vi "EminemStateMachine.vi"(5 "EminemCommand":bool[](array[boolean]), 7 "EminemCancel":bool, 8 "LowerShoot_At_Speed":bool, 9 "UpperShoot_At_Speed":bool, 10 "LowerShoot_Speed_RPM":dbl=1.0 format="%#_13g", 11 "UpperShoot_Speed_RPM":dbl=4000.0 format="%#_13g") -> (0 "Box states":T1=enum."13-AmpDone", 1 "AmpAndFeed-MotorDmd":dbl, 2 "LowerShooter-RPM_Dmd":dbl, 3 "UpperShooterAndAmp-RPM_Dmd":dbl)   [LabVIEW 2023]
doc: "Process Intake State Machine"
uses:
  Intake/IntakeState.ctl
  EminemStatesEnum.ctl
  _UNUSED/EminemNoteState.ctl
  <vilib>/Rock Robotics/WPI/ThirdParty/JAS_Junk/TrajLib/Trajectory_Library.lvlib
  EminemGlobals.vi
panel:
  in  "ActualShooterSpd":dbl
  # "WHAT IS THIS ???"
  # "Click here to set min"
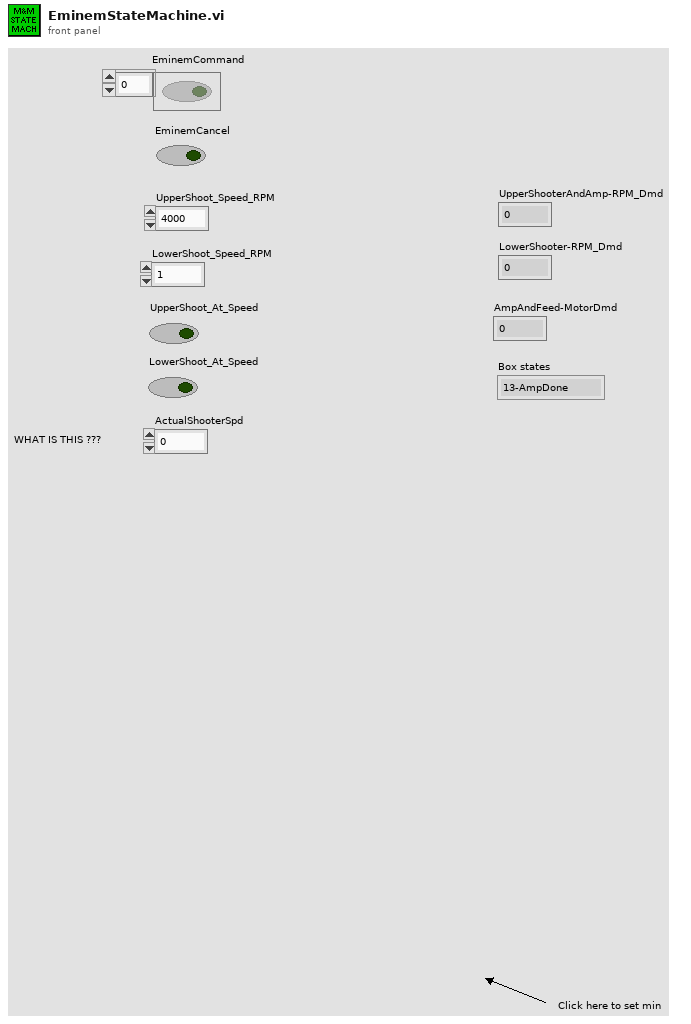
[diagram p1: front panel]
types:
  T1 = typedef "EminemStatesEnum.ctl" = enum16{"0-Init", "1-WaitForCmd", "2-Cancel", "3-ShootStart", "4-ShootRev", "5-ShootUpToSpd?", "6-ShootStartFeed&Timer", "7-ShootTimerOrSensorDone", "8-ShootDone", "9-AmpStart", "10-AmpUpToSpd?", "11-AmpStartFeed&Timer", "12-AmpTimerOrSensorDone", "13-AmpDone"}
  T2 = typedef "EminemNoteState.ctl" = enum16{"0-NoteInShooterWheels", "1-MisalignedNote", "2-NoNote", "3-HaveNote"}
  T3 = typedef "EminemStatesEnum.ctl" = enum16{"get input", "start shoot wheels", "up to speed?", "run intake", "have ring?", "stop intake and shooter", "start intake", "pick up ring or  _ sec?", "stop intake", "start source  intake", "pick up note?", "stop intake shooter", "shoot amp", "used note?", "stop amp intake", "initilization", "pre rev"}
  T4 = typedef "Trajectory_Library.lvlib/TIMER.ctl" = cluster{"StartTime":dbl, "Accumulated TIme":dbl, "Running":bool, "semaphore":T5}
  T5 = typedef "Semaphore RefNum" = refnum<k1>
  T6 = typedef "IntakeState.ctl" = enum16{"0-init", "1-cancel", "2-wait-for-cmd", "3-intake-check-for-note", "4-intake-start-intake", "5-intake-have-note-yet", "6-intake-stop-motor", "7-spit-out", "8-feed-note-to-shooter"}
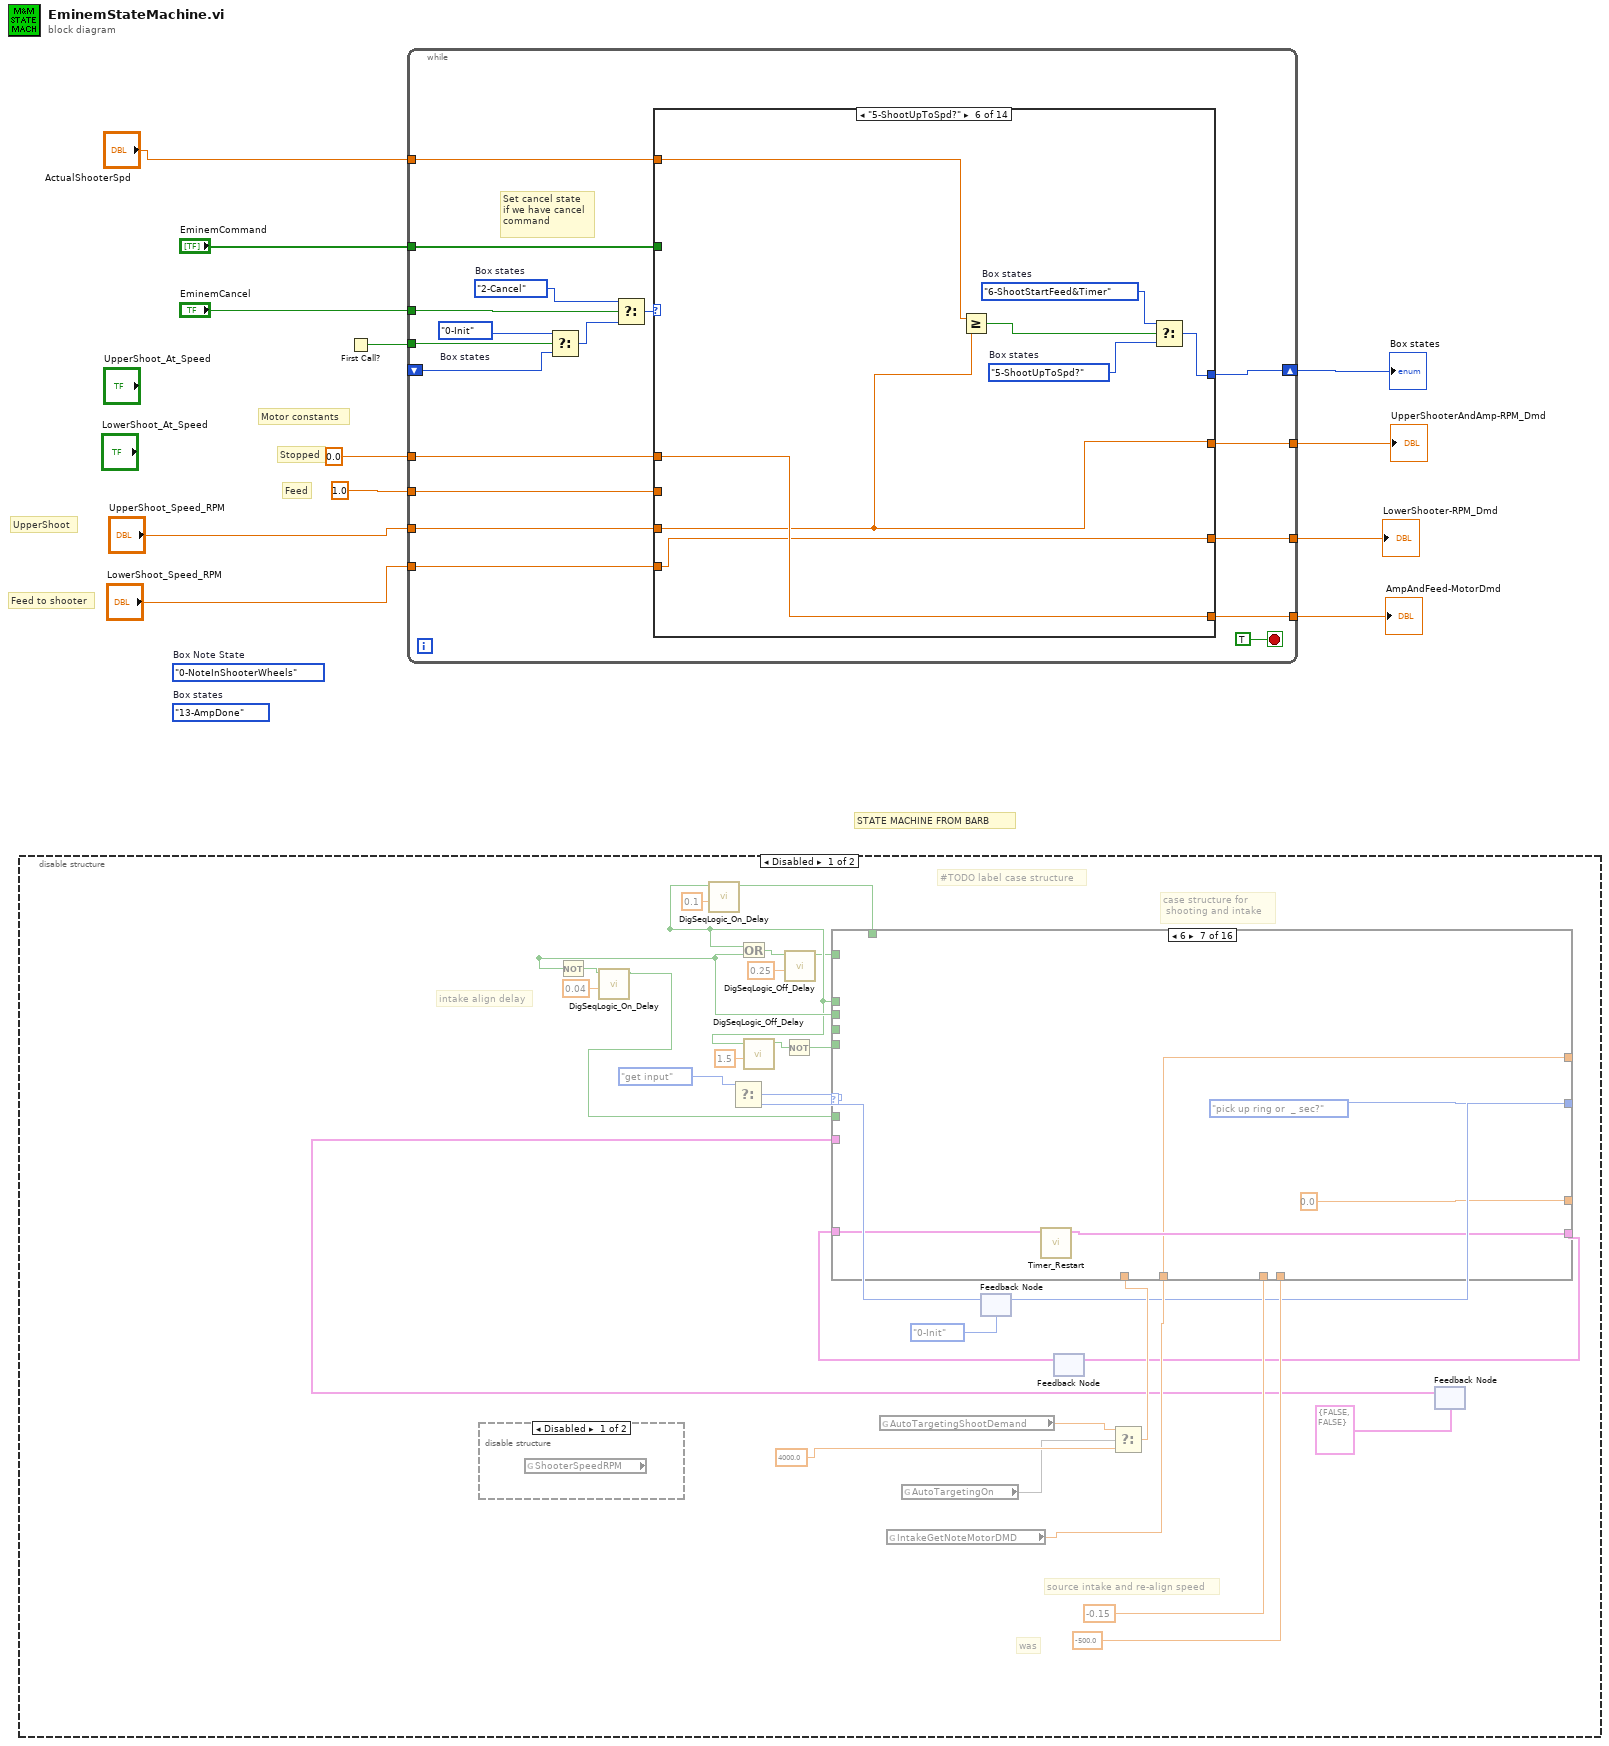
[diagram p0: block diagram]
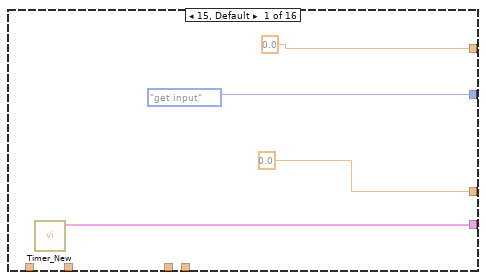
[diagram p3: hidden frame]
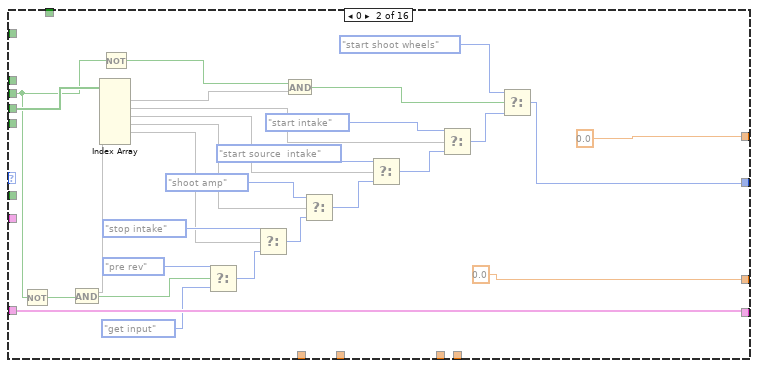
[diagram p4: hidden frame]
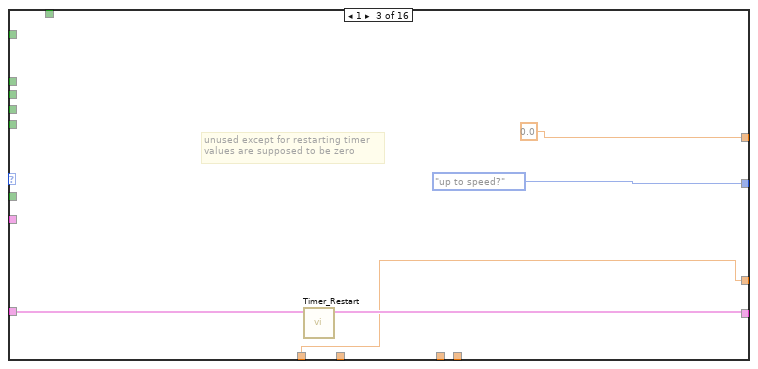
[diagram p5: hidden frame]
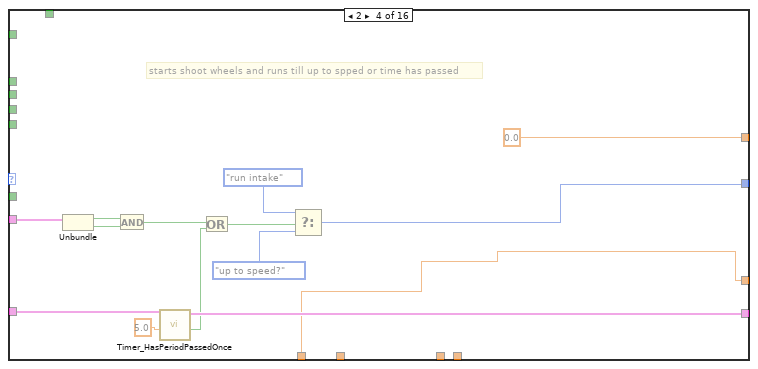
[diagram p6: hidden frame]
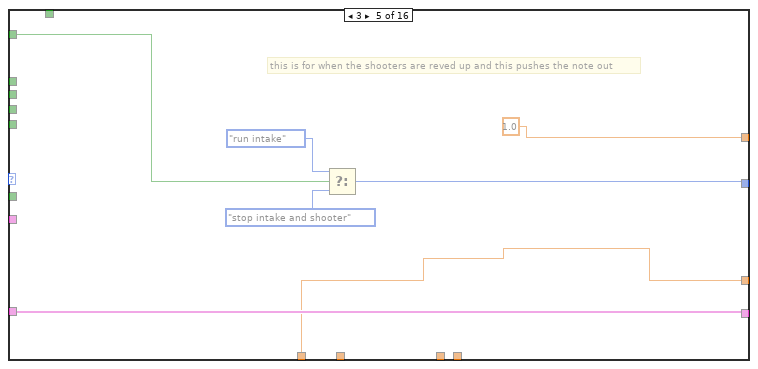
[diagram p7: hidden frame]
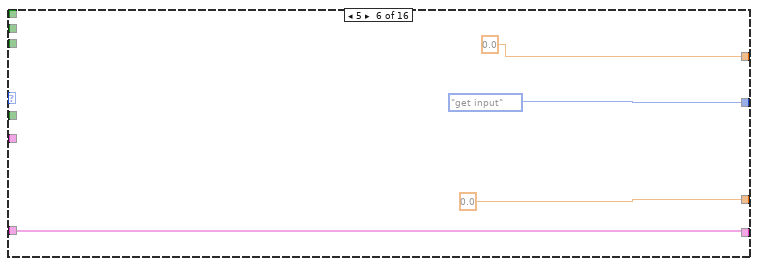
[diagram p8: hidden frame]
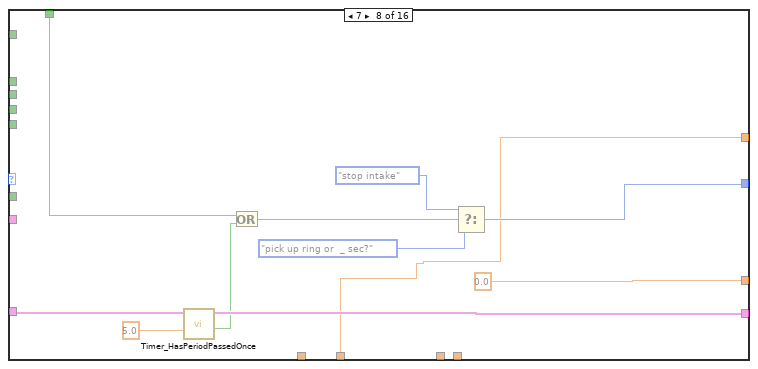
[diagram p9: hidden frame]
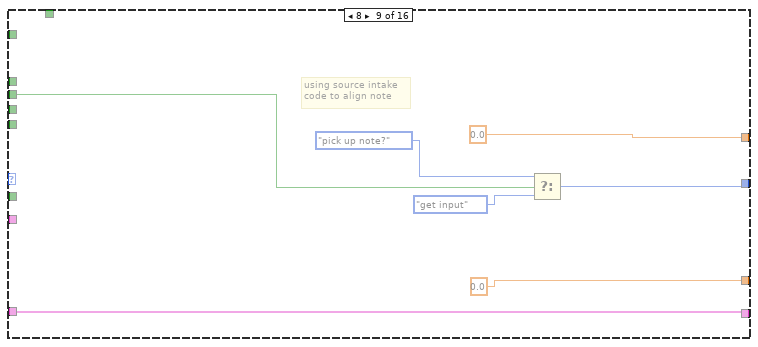
[diagram p10: hidden frame]
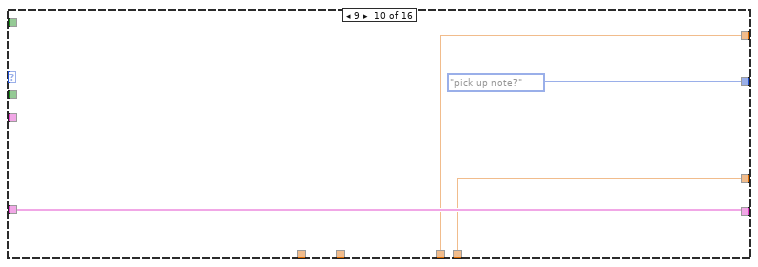
[diagram p11: hidden frame]
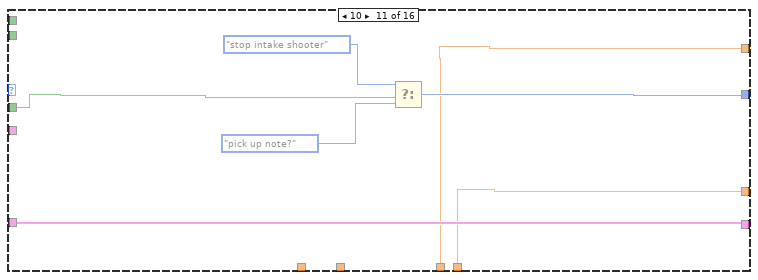
[diagram p12: hidden frame]
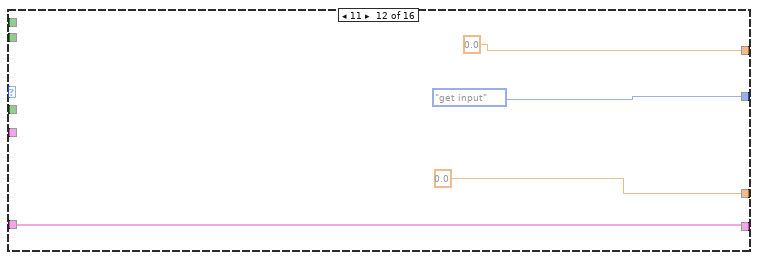
[diagram p13: hidden frame]
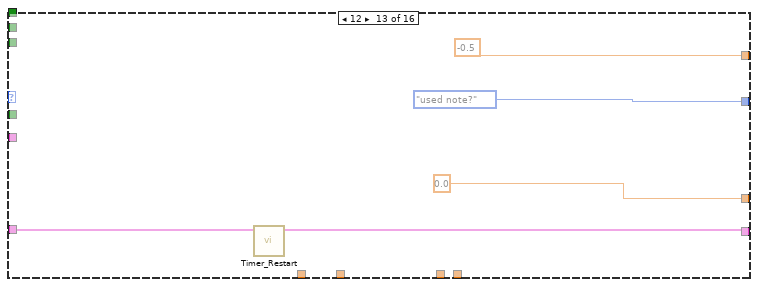
[diagram p14: hidden frame]
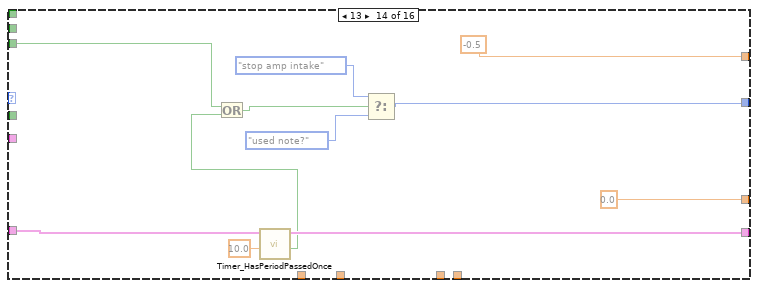
[diagram p15: hidden frame]
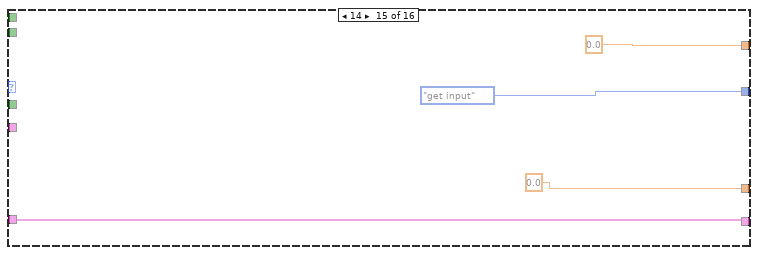
[diagram p16: hidden frame]
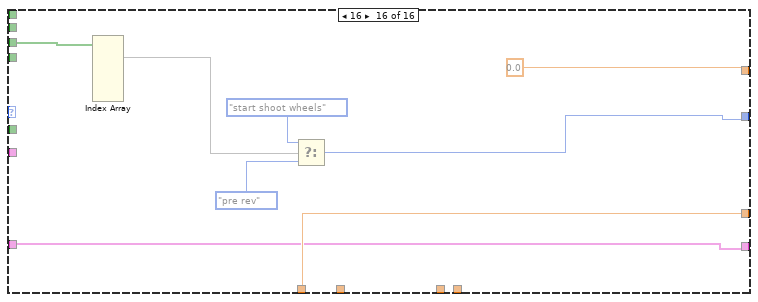
[diagram p17: hidden frame]
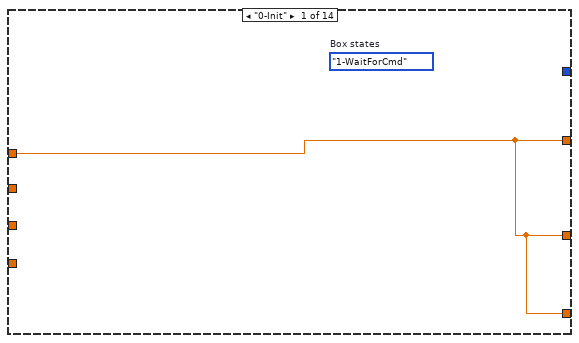
[diagram p19: hidden frame]
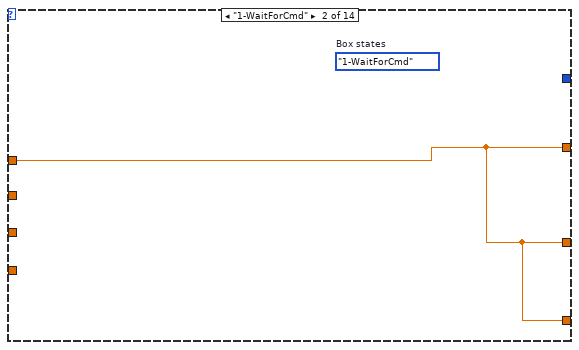
[diagram p20: hidden frame]
diagram:
  (unwired) EminemNoteState."0-NoteInShooterWheels"  # Box Note State
  (unwired) EminemStatesEnum."13-AmpDone"  # Box states
  # "STATE MACHINE FROM BARB"
  # "Feed to shooter"
  # "UpperShoot"
  # "Feed"
  # "Stopped"
  # "Motor constants"
  n1 = disable-structure shown="Disabled" {
    frame Disabled {
      # "intake align delay"
      # "was"
      # "source intake and re-align speed"
      # "#TODO label case structure"
      # "case structure for\n shooting and intake"
      n2 = disable-structure shown="Disabled" {
        frame Disabled {
          n3 = global read "EminemGlobals.vi" "ShooterSpeedRPM"() -> ()  [unwired: 1 out]
        }
        frame Enabled {
        }
      }
      n4 = global read "EminemGlobals.vi" "AutoTargetingShootDemand"() -> (w32:dbl)
      n5 = global read "EminemGlobals.vi" "IntakeGetNoteMotorDMD"() -> (w29:dbl)
      n6 = global read "EminemGlobals.vi" "AutoTargetingOn"() -> (w33)
      n7 = feedback #1(EminemStatesEnum."0-Init") -> (w38:u16)
      n8 = Select(t=EminemStatesEnum."get input" ("Box states"), f=w38) -> (s=w18:bool, s? t:f=w17:u16)
      n9 = feedback #2() -> (w22:T4)  [unwired: 1 in]
      n10 = Select(t=w32, s=w33, f=4000.0) -> (s? t:f=w34:dbl)
      n11 = feedback #3(cluster{bool, bool} {FALSE, FALSE}) -> (w15:cluster{bool, bool})
      n12 = feedback-in #3() -> ()  [unwired: 1 out]
      n13 = Not(x=w41) -> (.not. x?=w39:bool)
      n14 = call <vilib>:"DigSeqLogic_On_Delay.vi"("Delay"=0.04, "Input"=w39) -> ("Output"=w42:bool)  [unwired: 8 in, 1 out]
      n15 = call <vilib>:"DigSeqLogic_On_Delay.vi"("Delay"=0.1 ("On Delay Time\nSeconds"), "Input"=w35) -> ("Output"=w31:bool)  [unwired: 8 in, 1 out]
      n16 = Or(x=w35, y=w41) -> (x .or. y?=w24:bool)
      n17 = call <vilib>:"DigSeqLogic_Off_Delay.vi"("Delay"=0.25 ("Off Delay Tme\nSeconds"), "Input"=w24) -> ("Output"=w25:bool)  [unwired: 8 in, 1 out]
      n18 = call <vilib>:"DigSeqLogic_Off_Delay.vi"("Delay"=1.5 ("Off Delay Tme\nSeconds"), "Input"=w35) -> ("Output"=w27:bool)  [unwired: 8 in, 1 out]
      n19 = Not(x=w27) -> (.not. x?=w28:bool)
      n20 = case shown="6" w17 {
        tunnel: [EminemStatesEnum."get input" ("Box states") w69 EminemStatesEnum."up to speed?" ("Box states") w89 w98 EminemStatesEnum."get input" ("Box states") EminemStatesEnum."pick up ring or  _ sec?" ("Box states") w118 w125 EminemStatesEnum."pick up note?" ("Box states") w136 EminemStatesEnum."get input" ("Box states") EminemStatesEnum."used note?" ("Box states") w155 EminemStatesEnum."get input" ("Box states") w168] -> w14
        tunnel: w15 -> [_ _ _ w92 _ _ _ _ _ _ _ _ _ _ _ _]
        tunnel: [0.0 0.0 w76 w81 w95 0.0 0.0 0.0 0.0 w129 w134 0.0 0.0 0.0 0.0 w169] -> _
        tunnel: [0.0 0.0 0.0 0.0 1.0 0.0 w106 w112 0.0 w130 w135 0.0 -0.5 -0.5 0.0 0.0] -> _
        tunnel: [_ w74 _ _ _ _ _ _ _ _ _ _ _ _ _ w166] -> w16
        tunnel: [_ _ _ _ _ _ _ _ _ _ _ _ _ _ _ _] -> w35
        tunnel: [_ w51 _ _ _ _ _ _ w122 _ _ _ _ _ _ _] -> w41
        tunnel: [w44 w61 w77 w86 w97 w102 w108 w114 w126 w131 w139 w140 w144 w153 w160 w167] -> w21
        tunnel: w22 -> [_ w61 w78 w87 w97 w102 w107 w116 w126 w131 w139 w140 w145 w154 w160 w167]
        tunnel: w25 -> [_ _ _ _ w96 _ _ _ _ _ _ _ _ _ _ _]
        tunnel: w28 -> [_ _ _ _ _ _ _ _ _ _ _ _ _ w149 _ _]
        tunnel: w34 -> [_ _ w76 w81 w95 _ _ _ _ _ _ _ _ _ _ w169]
        tunnel: w29 -> [_ _ _ _ _ _ w106 w112 _ _ _ _ _ _ _ _]
        tunnel: w31 -> [_ _ _ _ _ _ _ w111 _ _ _ _ _ _ _ _]
        tunnel: -0.15 -> [_ _ _ _ _ _ _ _ _ w130 w135 _ _ _ _ _]
        tunnel: -500.0 -> [_ _ _ _ _ _ _ _ _ w129 w134 _ _ _ _ _]
        tunnel: w42 -> [_ _ _ _ _ _ _ _ _ _ w133 _ _ _ _ _]
        frame 15, Default {
          n21 = call <vilib>:"Timer_New.vi"() -> ("TIMER"=w44:T4)  [unwired: 11 in]
        }
        frame 0 {
          n22 = Not(x=w51) -> (.not. x?=w49:bool)
          n23 = Index Array(array=w74) -> (element #1=w59, element #2=w66, element #3=w65, element #4=w64, element #5=w55, element #6=w50)  [unwired: 6 in]
          n24 = And(x=w50, y=w49) -> (x .and. y?=w48:bool)
          n25 = Not(x=w51) -> (.not. x?=w58:bool)
          n26 = Select(t=EminemStatesEnum."pre rev" ("Box states"), s=w48, f=EminemStatesEnum."get input" ("Box states")) -> (s? t:f=w54:T3)
          n27 = Select(t=EminemStatesEnum."stop intake" ("Box states"), s=w55, f=w54) -> (s? t:f=w57:T3)
          n28 = And(x=w58, y=w59) -> (x .and. y?=w60:bool)
          n29 = Select(t=EminemStatesEnum."shoot amp" ("Box states"), s=w64, f=w57) -> (s? t:f=w70:T3)
          n30 = Select(t=EminemStatesEnum."start source  intake", s=w65, f=w70) -> (s? t:f=w71:T3)
          n31 = Select(t=EminemStatesEnum."start intake" ("Box states"), s=w66, f=w71) -> (s? t:f=w72:T3)
          n32 = Select(t=EminemStatesEnum."start shoot wheels" ("Box states"), s=w60, f=w72) -> (s? t:f=w69:T3)
        }
        frame 1 {
          # "unused except for restarting timer\nvalues are supposed to be zero"
          n33 = call <vilib>:"Timer_Restart.vi"("in Timer"=w78) -> ("out Timer"=w77:T4)  [unwired: 10 in]
        }
        frame 2 {
          # "starts shoot wheels and runs till up to spped or time has passed"
          n34 = Unbundle(w92) -> (w91:bool, w90:bool)
          n35 = And(x=w91, y=w90) -> (x .and. y?=w84:bool)
          n36 = call <vilib>:"Timer_HasPeriodPassedOnce.vi"("Period"=5.0, "in Timer"=w87) -> ("Expired"=w82:bool, "out Timer"=w86:T4)  [unwired: 7 in, 1 out]
          n37 = Or(x=w84, y=w82) -> (x .or. y?=w83:bool)
          n38 = Select(t=EminemStatesEnum."run intake" ("Box states"), s=w83, f=EminemStatesEnum."up to speed?" ("Box states")) -> (s? t:f=w89:T3)
        }
        frame 3 {
          # "this is for when the shooters are reved up and this pushes the note out"
          n39 = Select(t=EminemStatesEnum."run intake" ("Box states"), s=w96, f=EminemStatesEnum."stop intake and shooter" ("Box states")) -> (s? t:f=w98:T3)
        }
        frame 5 {
        }
        frame 6 {
          n40 = call <vilib>:"Timer_Restart.vi"("in Timer"=w107) -> ("out Timer"=w108:T4)  [unwired: 10 in]
        }
        frame 7 {
          n41 = call <vilib>:"Timer_HasPeriodPassedOnce.vi"("Period"=5.0, "in Timer"=w116) -> ("Expired"=w113:bool, "out Timer"=w114:T4)  [unwired: 7 in, 1 out]
          n42 = Or(x=w111, y=w113) -> (x .or. y?=w117:bool)
          n43 = Select(t=EminemStatesEnum."stop intake" ("Box states"), s=w117, f=EminemStatesEnum."pick up ring or  _ sec?" ("Box states")) -> (s? t:f=w118:T3)
        }
        frame 8 {
          # "using source intake \ncode to align note"
          n44 = Select(t=EminemStatesEnum."pick up note?" ("Box states"), s=w122, f=EminemStatesEnum."get input" ("Box states")) -> (s? t:f=w125:T3)
        }
        frame 9 {
        }
        frame 10 {
          n45 = Select(t=EminemStatesEnum."stop intake shooter" ("Box states"), s=w133, f=EminemStatesEnum."pick up note?" ("Box states")) -> (s? t:f=w136:T3)
        }
        frame 11 {
        }
        frame 12 {
          n46 = call <vilib>:"Timer_Restart.vi"("in Timer"=w145) -> ("out Timer"=w144:T4)  [unwired: 10 in]
        }
        frame 13 {
          n47 = call <vilib>:"Timer_HasPeriodPassedOnce.vi"("Period"=10.0, "in Timer"=w154) -> ("Expired"=w151:bool, "out Timer"=w153:T4)  [unwired: 7 in, 1 out]
          n48 = Or(x=w149, y=w151) -> (x .or. y?=w150:bool)
          n49 = Select(t=EminemStatesEnum."stop amp intake" ("Box states"), s=w150, f=EminemStatesEnum."used note?" ("Box states")) -> (s? t:f=w155:T3)
        }
        frame 14 {
        }
        frame 16 {
          n50 = Index Array(array=w166) -> (element #1=w164)  [unwired: 6 in, 5 out]
          n51 = Select(t=EminemStatesEnum."start shoot wheels" ("Box states"), s=w164, f=EminemStatesEnum."pre rev" ("Box states")) -> (s? t:f=w168:T3)
        }
      }
      n52 = feedback-in #1(w14) -> ()
      n53 = feedback-in #2(w21) -> ()
    }
    frame Enabled {
    }
  }
  n54 = First Call?() -> (First Call?: T/F=w9:bool)
  n55 = while {
    tunnel: "EminemCommand" -> [w189]
    tunnel: [w188] -> w11
    tunnel: "EminemCancel" -> [w185]
    shift-right: [w173] -> w2
    shift-left: _ -> [w182]
    tunnel: w9 -> [w183]
    tunnel: "LowerShoot_Speed_RPM" -> [w181]
    tunnel: "UpperShoot_Speed_RPM" -> [w180]
    tunnel: 1.0 -> [w179]
    tunnel: 0.0 -> [w178]
    tunnel: [w175] -> w4
    tunnel: [w174] -> w3
    tunnel: "ActualShooterSpd" -> [w172]
    stop <- TRUE stop-if-true
    w176 = EminemStatesEnum."0-Init"  # Box states
    w177 = EminemStatesEnum."2-Cancel"  # Box states
    # "Set cancel state\nif we have cancel\ncommand"
    n56 = Select(t=w176, s=w183, f=w182) -> (s? t:f=w184:T1)
    n57 = Select(t=w177, s=w185, f=w184) -> (s? t:f=w187:T1)
    n58 = case shown="\"5-ShootUpToSpd?\"" w187 {
      tunnel: [w190 w191 w193 w197 w198 w200 w207 w208 w209 _ _ _ _ _] -> w188
      tunnel: w189 -> [_ _ _ _ _ _ _ _ _ _ _ _ _ _]
      tunnel: w179 -> [_ _ _ _ w198 _ _ _ _ _ _ _ _ _]
      tunnel: w178 -> [w190 w191 w193 w195 _ w206 w207 _ _ _ _ _ _ _]
      tunnel: w180 -> [_ _ _ w197 _ w200 _ w208 _ _ _ _ _ _]
      tunnel: w181 -> [_ _ _ w196 _ w205 _ _ w209 _ _ _ _ _]
      tunnel: [w190 w191 w193 w196 _ w205 w207 _ _ _ _ _ _ _] -> w175
      tunnel: [w190 w191 w193 w195 _ w206 w207 _ _ _ _ _ _ _] -> w174
      tunnel: [_ _ w192 EminemStatesEnum."5-ShootUpToSpd?" ("Box states") _ w202 _ _ _ _ _ _ _ _] -> w173
      tunnel: w172 -> [_ _ _ _ _ w199 _ _ _ _ _ _ _ _]
      frame "0-Init" {
        (unwired) EminemStatesEnum."1-WaitForCmd"  # Box states
      }
      frame "1-WaitForCmd" {
        (unwired) EminemStatesEnum."1-WaitForCmd"  # Box states
      }
      frame "2-Cancel" {
        w192 = EminemStatesEnum."1-WaitForCmd"  # Box states
      }
      frame "3-ShootStart" {
        # "Cant intake if we already have a note !!!!"
      }
      frame "4-ShootRev" {
        (unwired) IntakeState."5-intake-have-note-yet" ("Box Note State")
      }
      frame "5-ShootUpToSpd?" {
        w203 = EminemStatesEnum."5-ShootUpToSpd?"  # Box states
        w204 = EminemStatesEnum."6-ShootStartFeed&Timer"  # Box states
        n59 = Greater Or Equal?(x=w199, y=w200) -> (x >= y?=w201:bool)
        n60 = Select(t=w204, s=w201, f=w203) -> (s? t:f=w202:T1)
      }
      frame "6-ShootStartFeed&Timer" {
        (unwired) EminemStatesEnum."1-WaitForCmd"  # Box states
      }
      frame "7-ShootTimerOrSensorDone" {
      }
      frame "8-ShootDone" {
      }
      frame "9-AmpStart" {
      }
      frame "10-AmpUpToSpd?" {
      }
      frame "11-AmpStartFeed&Timer" {
      }
      frame "12-AmpTimerOrSensorDone" {
      }
      frame "13-AmpDone" {
      }
    }
  }
  "UpperShooterAndAmp-RPM_Dmd" <- w11
  "AmpAndFeed-MotorDmd" <- w3
  "LowerShooter-RPM_Dmd" <- w4
  "Box states" <- w2
